vi "TSlIN TransmitHeader&Receive.vi"(0 "路径输入":path, 1 "ALINIdxchn":u8(ring) items=["CHN1", "CHN2", "CHN3", "CHN4", "CHN5", "CHN6", "CHN7", "CHN8", "CHN9", "CHN10", "CHN11", "CHN12", "CHN13", "CHN14", "CHN15", "CHN16", "CHN17", "CHN18", "CHN19", "CHN20", "CHN21", "CHN22", "CHN23", "CHN24", "CHN25", "CHN26", "CHN27", "CHN28", "CHN29", "CHN30", "CHN31", "CHN32"], 2 "ALINDLC":u8, 3 "ALINId":u32 format="%.0x") -> (4 "路径输出":path, 13 "ReceiveData":T1)   [LabVIEW 2013]
panel:
  out "错误输出":errorcluster
  in  "错误输入（无错误）":errorcluster
  out "tsapp_transmit_header_and_receive_msg":i32
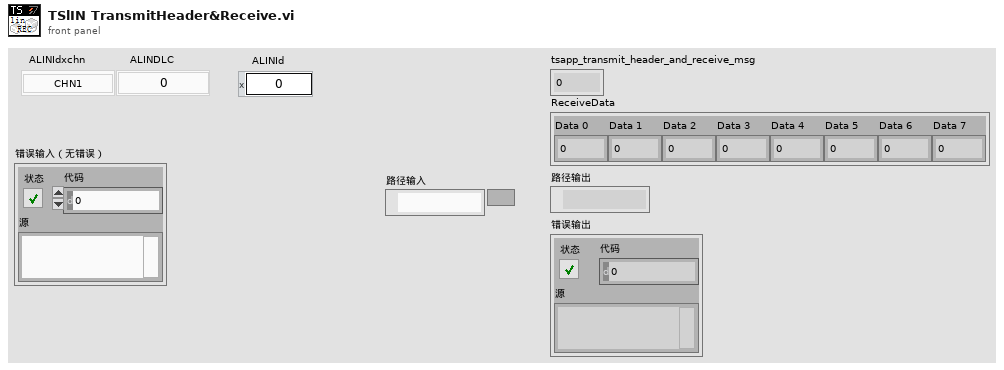
[diagram p1: front panel]
types:
  T1 = cluster{"Data 0":u8, "Data 1":u8, "Data 2":u8, "Data 3":u8, "Data 4":u8, "Data 5":u8, "Data 6":u8, "Data 7":u8}
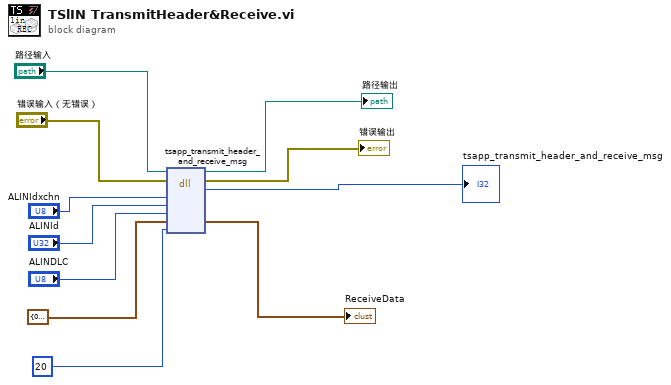
[diagram p0: block diagram]
diagram:
  n1 = dll-call lib="C:/Users/aa/Desktop/TSDemo/TSCAN_Labview_Demo_20220617_V1.25/Config/TSMaster.dll" fn="tsapp_transmit_header_and_receive_msg"(path in="路径输入", error in="错误输入（无错误）", "AChn"="ALINIdxchn", "AIdentifier"="ALINId", "ADLC"="ALINDLC", "簇"=T1 {"Data 0"=0, "Data 1"=0, "Data 2"=0, "Data 3"=0, "Data 4"=0, "Data 5"=0, "Data 6"=0, "Data 7"=0} ("ALINDataArray"), "ATimoutMS"=20) -> (path out=→"路径输出":path, error out=→"错误输出":errorcluster, "tsapp_transmit_header_and_receive_msg"=→"tsapp_transmit_header_and_receive_msg":i32, "簇"=→"ReceiveData":T1)  [unwired: 5 in]
